vi "Get Client Type.vi"(8 "error in (no error)":errorcluster, 11 "Instrument in":refnum<class "Instrument.lvclass">) -> (0 "error out":errorcluster, 2 "Client Type":T1, 3 "Instrument out":refnum<class "Instrument.lvclass">)   [LabVIEW 2019, in "Instrument.lvlib" / "Instrument.lvclass"]
uses:
  Instrument.lvclass
  Typedefs/Client Type--Enum.ctl
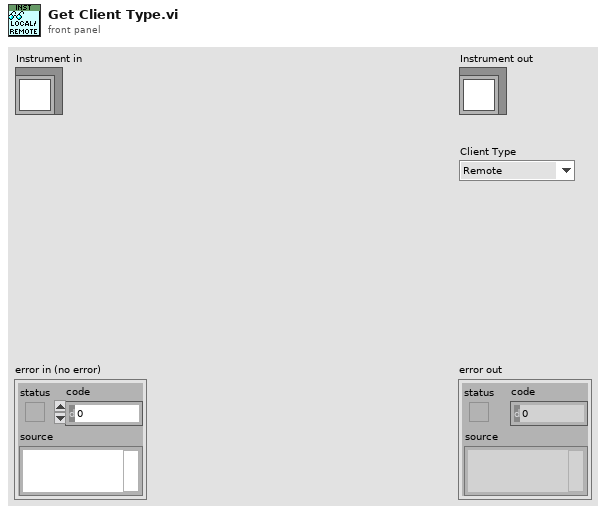
[diagram p1: front panel]
types:
  T1 = typedef "Instrument.lvlib/Instrument.lvclass/Client Type--Enum.ctl" = enum16{"Remote", "Local"}
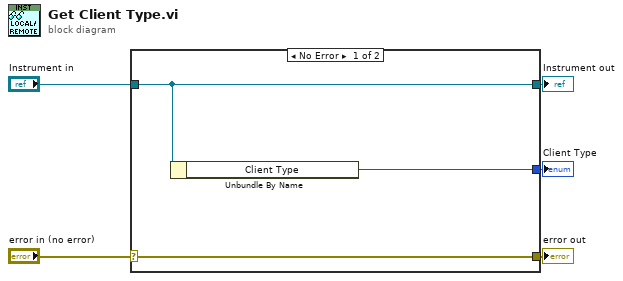
[diagram p0: block diagram]
diagram:
  n1 = case shown="No Error" "error in (no error)" {
    selector: "error in (no error)" -> [w8 w9]
    tunnel: [w8 w9] -> w4
    tunnel: [w7 w10] -> w2
    tunnel: "Instrument in" -> [w7 w10]
    tunnel: [w6 _] -> w1
    frame No Error {
      n2 = Unbundle By Name(w7) -> ("Client Type"=w6:T1)
    }
    frame Error {
    }
  }
  "error out" <- w4
  "Instrument out" <- w2
  "Client Type" <- w1
